vi "String to Item Text.vi"(11 "2D String Array":string[][](array[string])) -> (3 "Child Item Text":cluster{"2-D String":string[]}[](array[cluster]))   [LabVIEW 2022 SP3]
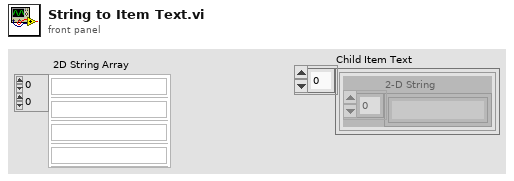
[diagram p1: front panel]
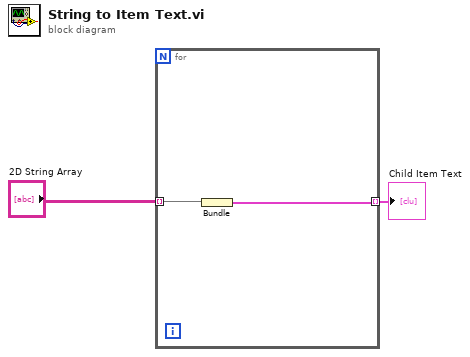
[diagram p0: block diagram]
diagram:
  n1 = for {
    tunnel: "2D String Array" -> [w4] mode=indexing
    tunnel: [w3] -> w2 mode=indexing
    n2 = Bundle("2D String Array"=w4) -> (w3:cluster{"2D String Array":string[]})  [unwired: 1 in]
  }
  "Child Item Text" <- w2
